vi "RS_RTO1024.vi"(4 "error in":T12, 7 "Command":string) -> (0 "error out":T12, 3 "Response":T10)   [LabVIEW 2018]
uses:
  MOKO_LabViewLibrary/MokoLowLevel/MokoLowLovelControl/MLLC_Error.ctl
  MOKO_LabViewLibrary/MokoLowLevel/MokoLowLovelControl/MLLC_Mode.ctl
  MOKO_LabViewLibrary/MokoLowLevel/MokoLowLovelControl/MLLC_Response.ctl
  MOKO_LabViewLibrary/MokoLowLevel/MokoLowLovelControl/MLLC_ConnectCluster.ctl
  MOKO_LabViewLibrary/MokoLowLevel/MokoLowLovelControl/MLLC_InterfaceType.ctl
  MOKO_LabViewLibrary/MokoLowLevel/MokoLowLovelControl/MLLC_OpenedSession.ctl
  MOKO_LabViewLibrary/MokoLowLevel/MokoLowLovelControl/MLLC_InterfaceSettings.ctl
  MOKO_LabViewLibrary/MokoLowLevel/MokoLowLovelControl/MLLC_InterfaceKind.ctl
  MOKO_LabViewLibrary/MokoLowLevel/MokoLowLovelControl/MLLC_DriverName.ctl
  MOKO_LabViewLibrary/MokoLowLevel/MokoLowLovelControl/MLLC_ErrorCode.ctl
  MOKO_LabViewLibrary/MokoLowLevel/MokoLowLovelControl/MLLC_ResponseInit.ctl
  MOKO_LabViewLibrary/MokoLowLevel/MokoLowLovelControl/MLLC_Request.ctl
  MOKO_LabViewLibrary/MokoLowLevel/MokoLowLovelControl/MLLC_Delay.ctl
panel:
  in  "Request":T1="*IDN?"
  in  "Response Init":T2="Rohde&Schwarz,FSW"
  in  "Error Code":T3=5450
  in  "Driver Name":T4="RS_RTO1024"
  in  "Settings":cluster{"Connect":T5}={"Connect"={"InterfaceType"=enum."VISA", "OpenedSession"="COM1", "InterfaceSettings"={"Interface"=enum."RS232", "EOS 4 read"=enum."LF (\\n)", "EOS 4 write"=enum."LF (\\n)", "TMO, ms"=10000, "Sett"=variant(cluster{"Baud Rate":u32, "Data Bits":u16, "Parity":u16, "Stop Bits":u16, "Flow Control":u16, "Eho":bool} {"Baud Rate"=75, "Data Bits"=0, "Parity"=0, "Stop Bits"=0, "Flow Control"=0, "Eho"=FALSE})}}}
  in  "Mode":T11=enum."Check"
  # "RS_RTO1024"
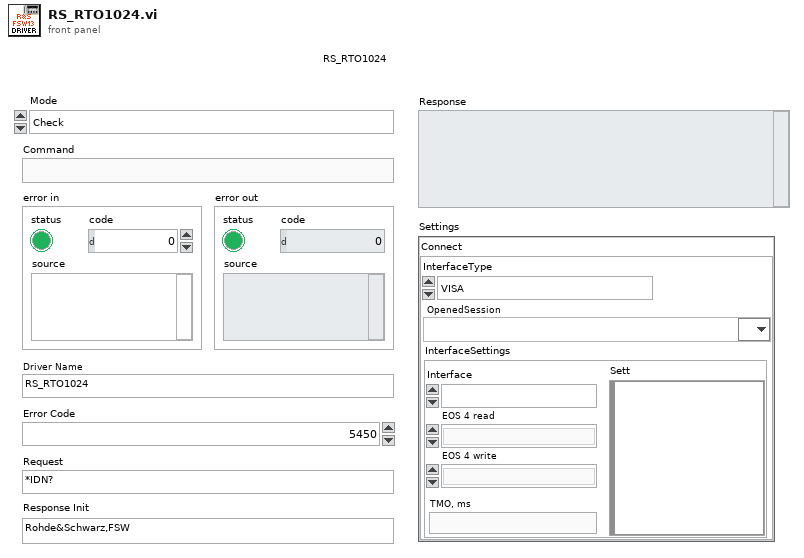
[diagram p1: front panel]
types:
  T1 = typedef "MLLC_Request.ctl" = string
  T2 = typedef "MLLC_ResponseInit.ctl" = string
  T3 = typedef "MLLC_ErrorCode.ctl" = u32
  T4 = typedef "MLLC_DriverName.ctl" = string
  T5 = typedef "MLLC_ConnectCluster.ctl" = cluster{"InterfaceType":T6, "OpenedSession":T7, "InterfaceSettings":T8}
  T6 = typedef "MLLC_InterfaceType.ctl" = enum16{"VISA", "Prologix USB-GPIB"}
  T7 = typedef "MLLC_OpenedSession.ctl" = refnum<visa-resource-name>
  T8 = typedef "MLLC_InterfaceSettings.ctl" = cluster{"Interface":T9, "EOS 4 read":enum16{"Default (=EOS 4 write)", "CR (\\r)", "LF (\\n)", "None"}, "EOS 4 write":enum16{"CR+LF (\\r\\n)", "CR (\\r)", "LF (\\n)", "None"}, "TMO, ms":i32, "Sett":variant}
  T9 = typedef "MLLC_InterfaceKind.ctl" = enum16{"RS232", "GPIB", "USB", "Ethernet", "another"}
  T10 = typedef "MLLC_Response.ctl" = string
  T11 = typedef "MLLC_Mode.ctl" = enum16{"get", "set", "close", "Init", "Check"}
  T12 = typedef "MLLC_Error.ctl" = errorcluster
  T13 = typedef "MLLC_Delay.ctl" = dbl
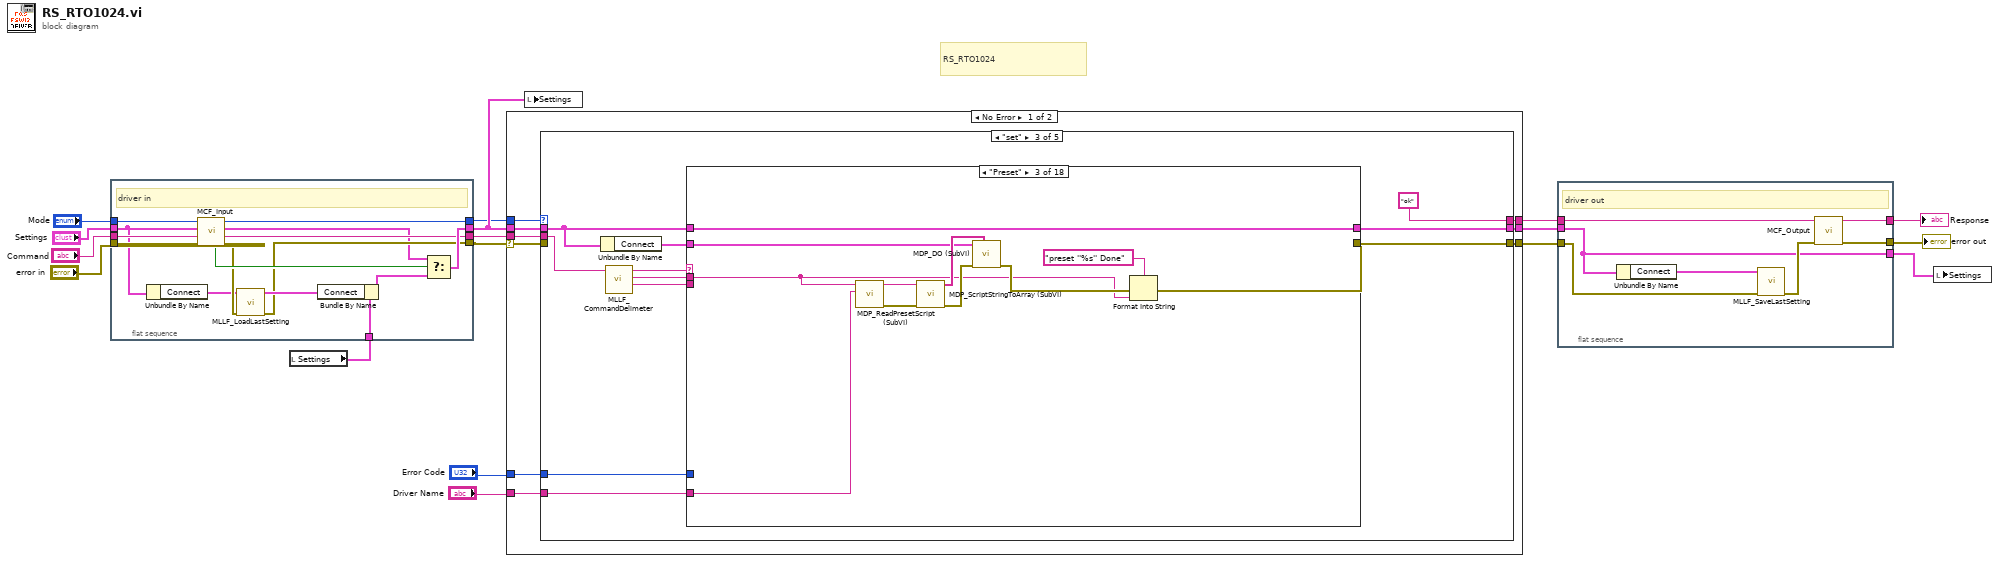
[diagram p0: block diagram]
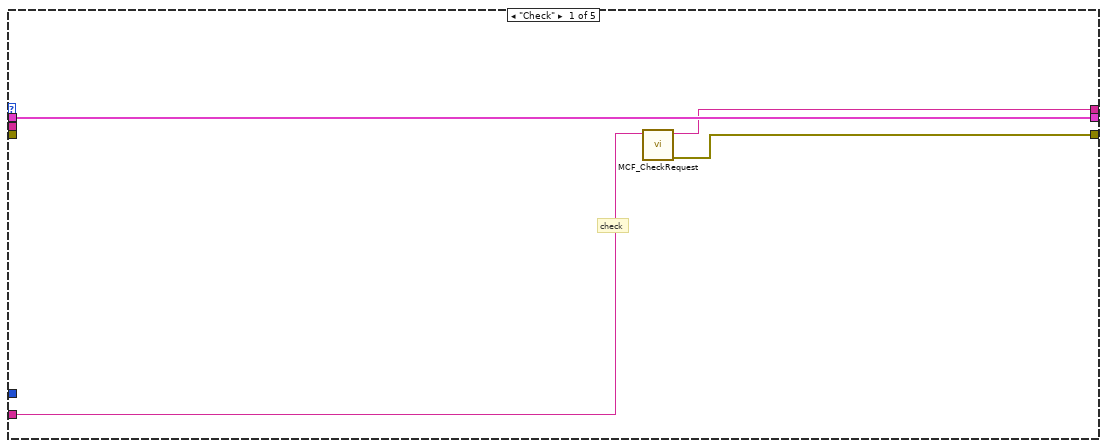
[diagram p2: hidden frame]
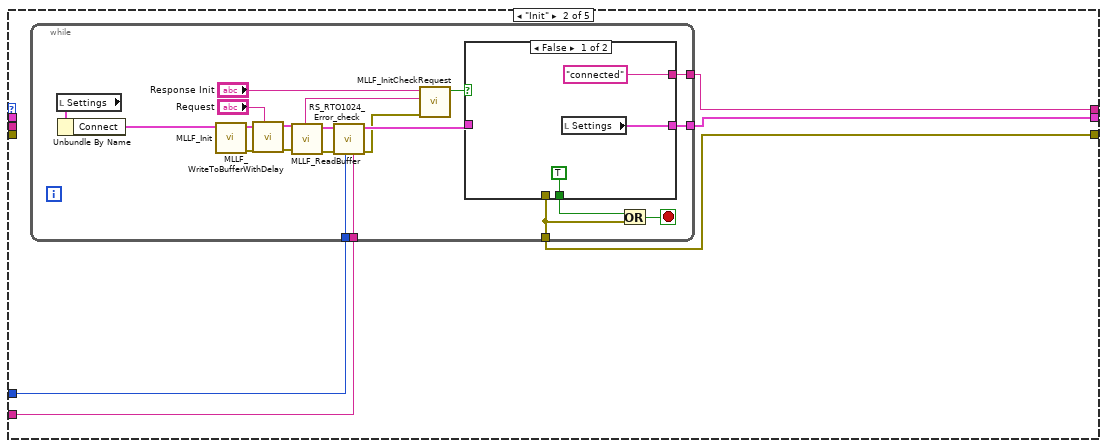
[diagram p3: hidden frame]
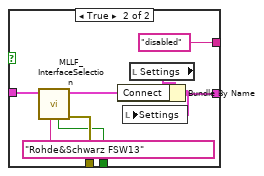
[diagram p4: hidden frame]
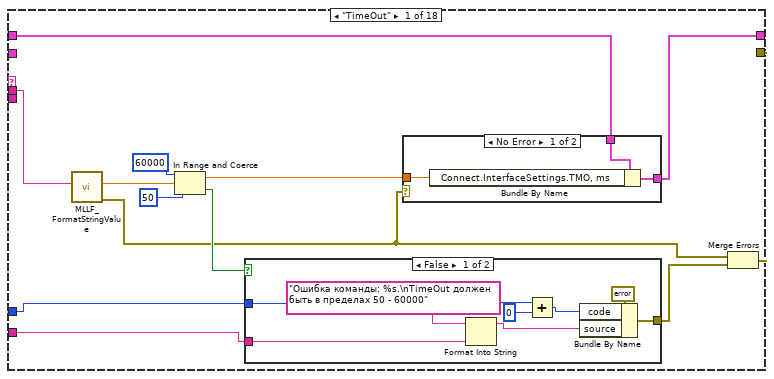
[diagram p5: hidden frame]
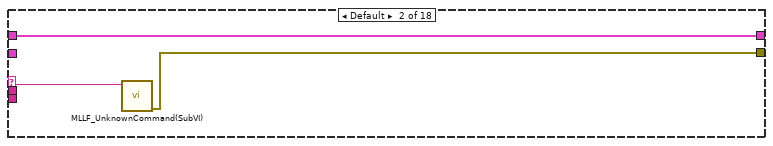
[diagram p8: hidden frame]
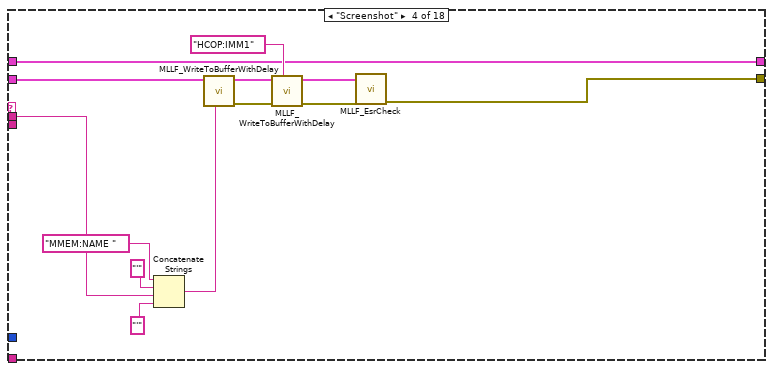
[diagram p9: hidden frame]
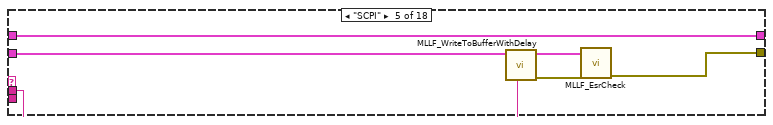
[diagram p10: hidden frame]
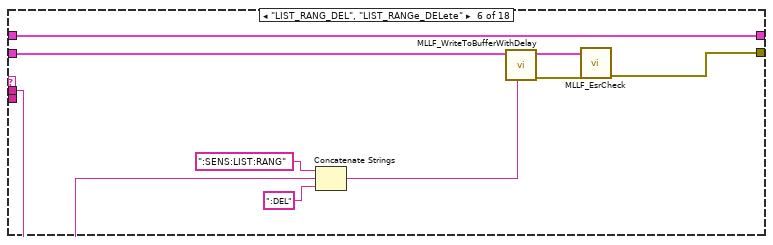
[diagram p11: hidden frame]
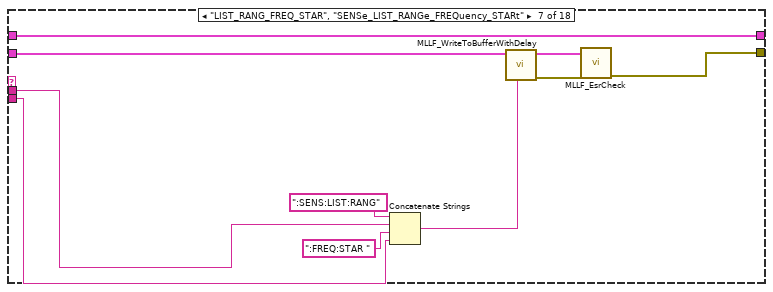
[diagram p12: hidden frame]
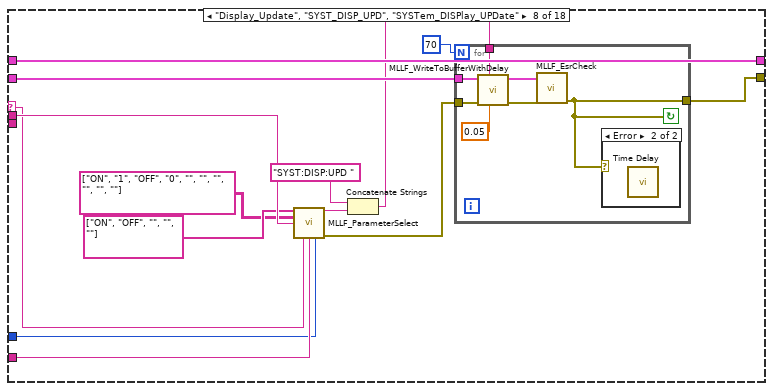
[diagram p13: hidden frame]
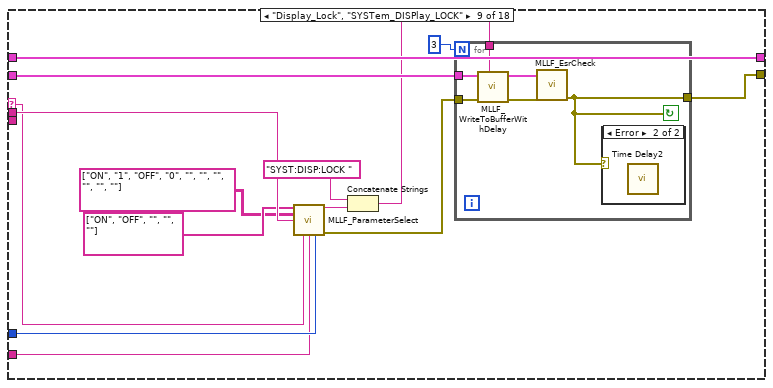
[diagram p15: hidden frame]
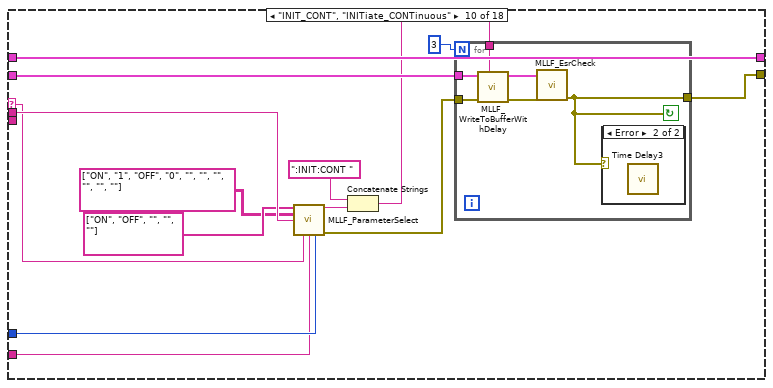
[diagram p17: hidden frame]
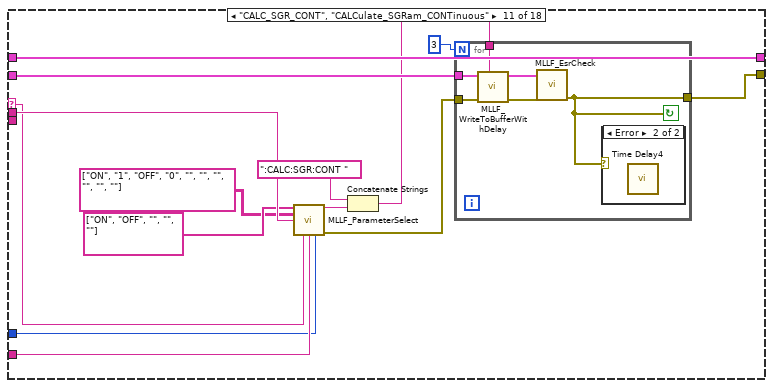
[diagram p19: hidden frame]
diagram:
  # "RS_RTO1024"
  n1 = flat-sequence {
    tunnel: [w22] -> w7
    tunnel: [w24] -> w8
    tunnel: "Command" -> [w25]
    tunnel: "Mode" -> [w27]
    tunnel: "Settings" -> [w19]
    tunnel: [w29] -> w10
    tunnel: w11 -> [w28]
    tunnel: "error in" -> [w21]
    tunnel: [w20] -> w9
    frame #0 {
      # "driver in"
      n2 = Unbundle By Name(w19) -> ("Connect"=w18:T5)
      n3 = call "MCF_Input.vi"("Error In"=w21, "Command in"=w25, "Mode in"=w27) -> ("Error Out"=w23:errorcluster, "Command out"=w24:string, "Mode out"=w20:T11, "Boolean"=w26:bool)  [unwired: 5 in]
      n4 = call "MLLF_LoadLastSetting.vi"("Error In"=w23, "DriverConnectCluster in"=w18) -> ("Error Out"=w22:errorcluster, "DriverConnectCluster out"=w30:T5)  [unwired: 8 in]
      n5 = Bundle By Name(cluster=w28, "Connect"=w30) -> (w31:cluster{"Connect":T5})
      n6 = Select(t=w19, s=w26, f=w31) -> (s? t:f=w29:cluster{"Connect":T5})
    }
  }
  n7 = local read "Settings"() -> (w11:cluster{"Connect":T5})
  n8 = case shown="No Error" w7 {
    selector: w7 -> [w36 w402]
    tunnel: [w38 w402] -> w1
    tunnel: w9 -> [w40 _]
    tunnel: [w39 "error" ("Output String")] -> w6
    tunnel: w8 -> [w37 _]
    tunnel: w10 -> [w33 w401]
    tunnel: "Error Code" -> [w35 _]
    tunnel: "Driver Name" -> [w34 _]
    tunnel: [w32 w401] -> w2
    frame No Error {
      n9 = case shown="\"set\"" w40 {
        tunnel: [w42 w47 "ok" ("Output String") w322 "close" ("Output String")] -> w39
        tunnel: [w41 w46 w85 w325 w398] -> w38
        tunnel: w37 -> [_ _ w92 w331 _]
        tunnel: w36 -> [_ _ _ _ _]
        tunnel: w35 -> [_ w49 w91 w328 _]
        tunnel: w34 -> [w43 w48 w88 w327 _]
        tunnel: w33 -> [w44 _ w90 w330 w397]
        tunnel: [w44 w45 w89 w329 w397] -> w32
        frame "Check" {
          # "check"
          # "Проверка подленности пользователя в соответствии с протоколом MD5."
          n10 = call "MCF_CheckRequest.vi"("Driver Name"=w43) -> ("Error Out"=w41:errorcluster, "Output String"=w42:string)  [unwired: 9 in]
        }
        frame "Init" {
          # "Тут проходит инициализация оборудования"
          n11 = while {
            tunnel: [w63] -> w46
            tunnel: w49 -> [w60]
            tunnel: w48 -> [w59]
            tunnel: [w55] -> w47
            tunnel: [w56] -> w45
            stop <- w62 stop-if-true
            n12 = local read "Settings"() -> (w66:cluster{"Connect":T5})
            n13 = Unbundle By Name(w66) -> ("Connect"=w52:T5)
            n14 = call "MLLF_Init.vi"("DriverConnect in"=w52) -> ("Error Out"=w68:errorcluster, "DriverConnect out"=w67:T5)  [unwired: 7 in]
            n15 = call "MLLF_WriteToBufferWithDelay.vi"("Command"="Request", "Error In"=w68, "DriverConnect in"=w67) -> ("Error Out"=w70:errorcluster, "DriverConnect out"=w69:T5)  [unwired: 7 in]
            n16 = call "MLLF_ReadBuffer.vi"("Error In"=w70, "DriverConnect in"=w69) -> ("Error Out"=w57:errorcluster, "DriverConnect out"=w58:T5, "String"=w54:string)  [unwired: 6 in]
            n17 = call "RS_RTO1024_Error_check.vi"("Driver Name"=w59, "Error Code"=w60, "error in"=w57, "DriverConnect in"=w58) -> ("error out"=w51:T12, "DriverConnect out"=w61:T5)  [unwired: 6 in]
            n18 = call "MLLF_InitCheckRequest.vi"("error in (no error)"=w51, "Answer"=w54, "Response Init"="Response Init") -> ("Design"=w50:bool)  [unwired: 5 in, 3 out]
            n19 = case shown="False" w50 {
              tunnel: w61 -> [_ w80]
              tunnel: [TRUE w74] -> w64
              tunnel: [_ w81] -> w63
              tunnel: [w72 w76] -> w56
              tunnel: ["connected" "disabled"] -> w55
              frame False {
                n20 = local read "Settings"() -> (w72:cluster{"Connect":T5})
              }
              frame True {
                n21 = call "MLLF_InterfaceSelection.vi"("Driver Name"="Rohde&Schwarz FSW13" ("String"), "DriverConnect in"=w80) -> ("error out"=w81:T12, "DriverConnect out"=w78:T5, "stop init?"=w74:bool)  [unwired: 5 in, 2 out]
                n22 = local read "Settings"() -> (w77:cluster{"Connect":T5})
                n23 = Bundle By Name(cluster=w77, "Connect"=w78) -> (w76:cluster{"Connect":T5})
                n24 = local write "Settings"(w76) -> ()
              }
            }
            n25 = Or(x=w64, y=w63) -> (x .or. y?=w62:bool)
          }
        }
        frame "set" {
          # "Тут реализованы функции DriverSet"
          n26 = Unbundle By Name(w90) -> ("Connect"=w86:T5)
          n27 = call "MLLF_CommandDelimeter.vi"("command with param"=w92) -> ("param 2"=w82:string, "param 1"=w83:string, "command"=w84:string)  [unwired: 6 in, 2 out]
          n28 = case shown="\"Preset\"" w84 {
            selector: w84 -> [_ w119 _ _ _ _ _ w170 w191 w211 w231 w251 _ _ _ _ _ _]
            tunnel: w90 -> [w95 w120 w121 w136 w149 w158 w168 w183 w204 w224 w244 w264 w275 w285 w299 w308 w314 w321]
            tunnel: [w94 w120 w121 w136 w149 w158 w168 w183 w204 w224 w244 w264 w275 w285 w299 w308 w314 w321] -> w89
            tunnel: w83 -> [w93 _ w124 w135 w147 w152 w161 w180 w201 w221 w241 w261 _ _ w292 _ _ _]
            tunnel: w91 -> [w97 _ _ _ _ _ _ w171 w193 w213 w232 w253 _ _ _ _ _ _]
            tunnel: w88 -> [w98 _ w123 _ _ _ _ w172 w192 w212 w233 w252 _ _ _ _ _ _]
            tunnel: [w96 w118 w122 w132 w148 w157 w167 w182 w203 w223 w243 w263 w274 w284 w298 w307 w313 w320] -> w85
            tunnel: w86 -> [_ _ w125 w144 w150 w159 w169 w181 w202 w222 w242 w262 w273 w283 w297 w306 w312 w319]
            tunnel: w82 -> [_ _ _ _ _ _ w160 _ _ _ _ _ _ _ w291 _ _ _]
            frame "TimeOut" {
              n29 = call "MLLF_FormatStringValue.vi"("String Value"=w93) -> ("error out"=w100:T12, "number"=w99:dbl)  [unwired: 8 in, 1 out]
              n30 = In Range and Coerce(upper limit=60000, x=w99, lower limit=50) -> (coerced(x)=w103:dbl, In Range?=w101:bool)
              n31 = case shown="False" w101 {
                tunnel: [w112 _] -> w102
                tunnel: w97 -> [w111 _]
                tunnel: w98 -> [w110 _]
                frame False {
                  n32 = Format Into String(format string="Ошибка команды: %s.\nTimeOut должен быть в пределах 50 - 60000", w110) -> (resulting string=w114:string)  [unwired: 2 in, 1 out]
                  n33 = Add(x=w111, y=0) -> (x+y=w115:T3)
                  n34 = Bundle By Name(cluster=errorcluster {"status"=TRUE, "code"=0, "source"=""} ("error out"), "code"=w115, "source"=w114) -> (w112:errorcluster)
                }
                frame True {
                }
              }
              n35 = case shown="No Error" w100 {
                tunnel: [w108 w109] -> w94
                tunnel: w95 -> [w107 w109]
                tunnel: w103 -> [w106 _]
                frame No Error {
                  n36 = Bundle By Name(cluster=w107, "Connect.InterfaceSettings.TMO, ms"=w106) -> (w108:cluster{"Connect":T5})
                }
                frame Error {
                }
              }
              n37 = Merge Errors(w100, w102) -> (w96:errorcluster)
            }
            frame Default {
              n38 = call "MLLF_UnknownCommand(SubVI).vi"("Unknown command"=w119) -> ("error out"=w118:errorcluster)  [unwired: 10 in]
            }
            frame "Preset" {
              n39 = call "MDP_ReadPresetScript (SubVI).vi"("Driver Name"=w123, "String in"=w124) -> ("Error Out"=w129:errorcluster, "String out"=w130:string)  [unwired: 8 in]
              n40 = call "MDP_ScriptStringToArray (SubVI).vi"("Error In"=w129, "String script"=w130) -> ("Error Out"=w131:errorcluster, "Array script"=w126:string[])  [unwired: 8 in]
              n41 = call "MDP_DO (SubVI).vi"("Array script"=w126, "Error in (no error)"=w131, "DriverConnect in"=w125) -> ("Error Out"=w127:errorcluster)  [unwired: 7 in, 1 out]
              n42 = Format Into String(format string="preset ''%s'' Done" ("Befor substring"), error in=w127, w124) -> (error out=w122:errorcluster)  [unwired: 1 in, 1 out]
            }
            frame "Screenshot" {
              n43 = Concatenate Strings("MMEM:NAME " ("String"), "'" ("string"), w135, "'" ("string")) -> (w139:string)
              n44 = call "MLLF_WriteToBufferWithDelay.vi"("Command"=w139, "DriverConnect in"=w144) -> ("Error Out"=w138:errorcluster, "DriverConnect out"=w143:T5)  [unwired: 8 in]
              n45 = call "MLLF_WriteToBufferWithDelay.vi"("Command"="HCOP:IMM1" ("String"), "Error In"=w138, "DriverConnect in"=w143) -> ("Error Out"=w134:errorcluster, "DriverConnect out"=w133:T5)  [unwired: 7 in]
              n46 = call "MLLF_EsrCheck.vi"("error in"=w134, "DriverConnect in"=w133) -> ("error out"=w132:T12)  [unwired: 8 in, 1 out]
            }
            frame "SCPI" {
              n47 = call "MLLF_WriteToBufferWithDelay.vi"("Command"=w147, "DriverConnect in"=w150) -> ("Error Out"=w145:errorcluster, "DriverConnect out"=w146:T5)  [unwired: 8 in]
              n48 = call "MLLF_EsrCheck.vi"("error in"=w145, "DriverConnect in"=w146) -> ("error out"=w148:T12)  [unwired: 8 in, 1 out]
            }
            frame "LIST_RANG_DEL", "LIST_RANGe_DELete" {
              n49 = Concatenate Strings(":SENS:LIST:RANG" ("String"), w152, ":DEL" ("string")) -> (w151:string)
              n50 = call "MLLF_WriteToBufferWithDelay.vi"("Command"=w151, "DriverConnect in"=w159) -> ("Error Out"=w155:errorcluster, "DriverConnect out"=w156:T5)  [unwired: 8 in]
              n51 = call "MLLF_EsrCheck.vi"("error in"=w155, "DriverConnect in"=w156) -> ("error out"=w157:T12)  [unwired: 8 in, 1 out]
            }
            frame "LIST_RANG_FREQ_STAR", "SENSe_LIST_RANGe_FREQuency_STARt" {
              n52 = Concatenate Strings(":SENS:LIST:RANG" ("String"), w161, ":FREQ:STAR " ("string"), w160) -> (w162:string)
              n53 = call "MLLF_WriteToBufferWithDelay.vi"("Command"=w162, "DriverConnect in"=w169) -> ("Error Out"=w165:errorcluster, "DriverConnect out"=w166:T5)  [unwired: 8 in]
              n54 = call "MLLF_EsrCheck.vi"("error in"=w165, "DriverConnect in"=w166) -> ("error out"=w167:T12)  [unwired: 8 in, 1 out]
            }
            frame "Display_Update", "SYST_DISP_UPD", "SYSTem_DISPlay_UPDate" {
              n55 = call "MLLF_ParameterSelect.vi"("Command to equipment"=string[] ["ON", "OFF", "", "", ""], "Names"=string[][] [["ON", "1"], ["OFF", "0"], ["", ""], ["", ""], ["", ""]], "Input"=w180, "Command"=w170, "Driver Name"=w172, "Error Code"=w171) -> ("Choice"=w176:string, "Error Out"=w173:errorcluster)  [unwired: 8 in]
              n56 = Concatenate Strings("SYST:DISP:UPD " ("string"), w176) -> (w175:string)
              n57 = for {
                N: 70 -> [_]
                tunnel: [w185] -> w182
                tunnel: w181 -> [w188]
                tunnel: w175 -> [w187]
                tunnel: w173 -> [w186]
                stop <- w185 continue-if-true
                n58 = call "MLLF_WriteToBufferWithDelay.vi"("Delay Time ( 0,05 s)"=T13 0.05, "Command"=w187, "Error In"=w186, "DriverConnect in"=w188) -> ("Error Out"=w190:errorcluster, "DriverConnect out"=w189:T5)  [unwired: 6 in]
                n59 = call "MLLF_EsrCheck.vi"("error in"=w190, "DriverConnect in"=w189) -> ("error out"=w185:T12)  [unwired: 8 in, 1 out]
                n60 = case shown="Error" w185 {
                  frame No Error {
                  }
                  frame Error {
                    n61 = call "Time Delay"() -> ()  [unwired: 11 in, 1 out]
                  }
                }
              }
            }
            frame "Display_Lock", "SYSTem_DISPlay_LOCK" {
              n62 = call "MLLF_ParameterSelect.vi"("Command to equipment"=string[] ["ON", "OFF", "", "", ""], "Names"=string[][] [["ON", "1"], ["OFF", "0"], ["", ""], ["", ""], ["", ""]], "Input"=w201, "Command"=w191, "Driver Name"=w192, "Error Code"=w193) -> ("Choice"=w197:string, "Error Out"=w194:errorcluster)  [unwired: 8 in]
              n63 = Concatenate Strings("SYST:DISP:LOCK " ("string"), w197) -> (w196:string)
              n64 = for {
                N: 3 -> [_]
                tunnel: [w205] -> w203
                tunnel: w202 -> [w208]
                tunnel: w196 -> [w207]
                tunnel: w194 -> [w206]
                stop <- w205 continue-if-true
                n65 = call "MLLF_WriteToBufferWithDelay.vi"("Command"=w207, "Error In"=w206, "DriverConnect in"=w208) -> ("Error Out"=w210:errorcluster, "DriverConnect out"=w209:T5)  [unwired: 7 in]
                n66 = call "MLLF_EsrCheck.vi"("error in"=w210, "DriverConnect in"=w209) -> ("error out"=w205:T12)  [unwired: 8 in, 1 out]
                n67 = case shown="Error" w205 {
                  frame No Error {
                  }
                  frame Error {
                    n68 = call "Time Delay2"() -> ()  [unwired: 11 in, 1 out]
                  }
                }
              }
            }
            frame "INIT_CONT", "INITiate_CONTinuous" {
              n69 = call "MLLF_ParameterSelect.vi"("Command to equipment"=string[] ["ON", "OFF", "", "", ""], "Names"=string[][] [["ON", "1"], ["OFF", "0"], ["", ""], ["", ""], ["", ""]], "Input"=w221, "Command"=w211, "Driver Name"=w212, "Error Code"=w213) -> ("Choice"=w217:string, "Error Out"=w214:errorcluster)  [unwired: 8 in]
              n70 = Concatenate Strings(":INIT:CONT " ("string"), w217) -> (w216:string)
              n71 = for {
                N: 3 -> [_]
                tunnel: [w225] -> w223
                tunnel: w222 -> [w228]
                tunnel: w216 -> [w227]
                tunnel: w214 -> [w226]
                stop <- w225 continue-if-true
                n72 = call "MLLF_WriteToBufferWithDelay.vi"("Command"=w227, "Error In"=w226, "DriverConnect in"=w228) -> ("Error Out"=w230:errorcluster, "DriverConnect out"=w229:T5)  [unwired: 7 in]
                n73 = call "MLLF_EsrCheck.vi"("error in"=w230, "DriverConnect in"=w229) -> ("error out"=w225:T12)  [unwired: 8 in, 1 out]
                n74 = case shown="Error" w225 {
                  frame No Error {
                  }
                  frame Error {
                    n75 = call "Time Delay3"() -> ()  [unwired: 11 in, 1 out]
                  }
                }
              }
            }
            frame "CALC_SGR_CONT", "CALCulate_SGRam_CONTinuous" {
              n76 = call "MLLF_ParameterSelect.vi"("Command to equipment"=string[] ["ON", "OFF", "", "", ""], "Names"=string[][] [["ON", "1"], ["OFF", "0"], ["", ""], ["", ""], ["", ""]], "Input"=w241, "Command"=w231, "Driver Name"=w233, "Error Code"=w232) -> ("Choice"=w237:string, "Error Out"=w234:errorcluster)  [unwired: 8 in]
              n77 = Concatenate Strings(":CALC:SGR:CONT " ("string"), w237) -> (w236:string)
              n78 = for {
                N: 3 -> [_]
                tunnel: [w245] -> w243
                tunnel: w242 -> [w248]
                tunnel: w236 -> [w247]
                tunnel: w234 -> [w246]
                stop <- w245 continue-if-true
                n79 = call "MLLF_WriteToBufferWithDelay.vi"("Command"=w247, "Error In"=w246, "DriverConnect in"=w248) -> ("Error Out"=w250:errorcluster, "DriverConnect out"=w249:T5)  [unwired: 7 in]
                n80 = call "MLLF_EsrCheck.vi"("error in"=w250, "DriverConnect in"=w249) -> ("error out"=w245:T12)  [unwired: 8 in, 1 out]
                n81 = case shown="Error" w245 {
                  frame No Error {
                  }
                  frame Error {
                    n82 = call "Time Delay4"() -> ()  [unwired: 11 in, 1 out]
                  }
                }
              }
            }
            frame "CALC_SPEC_CONT", "CALCulate_SPECtrogram_CONTinuous" {
              n83 = call "MLLF_ParameterSelect.vi"("Command to equipment"=string[] ["ON", "OFF", "", "", ""], "Names"=string[][] [["ON", "1"], ["OFF", "0"], ["", ""], ["", ""], ["", ""]], "Input"=w261, "Command"=w251, "Driver Name"=w252, "Error Code"=w253) -> ("Choice"=w257:string, "Error Out"=w254:errorcluster)  [unwired: 8 in]
              n84 = Concatenate Strings(":CALC:SPEC:CONT " ("string"), w257) -> (w256:string)
              n85 = for {
                N: 3 -> [_]
                tunnel: [w265] -> w263
                tunnel: w262 -> [w268]
                tunnel: w256 -> [w267]
                tunnel: w254 -> [w266]
                stop <- w265 continue-if-true
                n86 = call "MLLF_WriteToBufferWithDelay.vi"("Command"=w267, "Error In"=w266, "DriverConnect in"=w268) -> ("Error Out"=w270:errorcluster, "DriverConnect out"=w269:T5)  [unwired: 7 in]
                n87 = call "MLLF_EsrCheck.vi"("error in"=w270, "DriverConnect in"=w269) -> ("error out"=w265:T12)  [unwired: 8 in, 1 out]
                n88 = case shown="Error" w265 {
                  frame No Error {
                  }
                  frame Error {
                    n89 = call "Time Delay6"() -> ()  [unwired: 11 in, 1 out]
                  }
                }
              }
            }
            frame "CALC_SGR_CLE", "CALCulate_SGRam_CLEar" {
              n90 = for {
                N: 3 -> [_]
                tunnel: [w276] -> w274
                tunnel: w273 -> [w278]
                tunnel: "CALC:SGR:CLE" ("string") -> [w277]
                stop <- w276 continue-if-true
                n91 = call "MLLF_WriteToBufferWithDelay.vi"("Command"=w277, "DriverConnect in"=w278) -> ("Error Out"=w280:errorcluster, "DriverConnect out"=w279:T5)  [unwired: 8 in]
                n92 = call "MLLF_EsrCheck.vi"("error in"=w280, "DriverConnect in"=w279) -> ("error out"=w276:T12)  [unwired: 8 in, 1 out]
                n93 = case shown="Error" w276 {
                  frame No Error {
                  }
                  frame Error {
                    n94 = call "Time Delay7"() -> ()  [unwired: 11 in, 1 out]
                  }
                }
              }
            }
            frame "CALC_SPEC_CLE", "CALCulate_SPECtrogram_CLEar" {
              n95 = for {
                N: 3 -> [_]
                tunnel: [w286] -> w284
                tunnel: w283 -> [w288]
                tunnel: "CALC:SPEC:CLE" ("string") -> [w287]
                stop <- w286 continue-if-true
                n96 = call "MLLF_WriteToBufferWithDelay.vi"("Command"=w287, "DriverConnect in"=w288) -> ("Error Out"=w290:errorcluster, "DriverConnect out"=w289:T5)  [unwired: 8 in]
                n97 = call "MLLF_EsrCheck.vi"("error in"=w290, "DriverConnect in"=w289) -> ("error out"=w286:T12)  [unwired: 8 in, 1 out]
                n98 = case shown="Error" w286 {
                  frame No Error {
                  }
                  frame Error {
                    n99 = call "Time Delay8"() -> ()  [unwired: 11 in, 1 out]
                  }
                }
              }
            }
            frame "INIT_OPC", "INITiate_OPC" {
              n100 = case shown="\"Timeout\", \"TMO\"" w292 {
                tunnel: w291 -> [_ w302]
                tunnel: [20.0 w301] -> w293
                frame "False", Default {
                }
                frame "Timeout", "TMO" {
                  n101 = Scan From String(input string=w302) -> (output 1=w301:dbl)  [unwired: 4 in, 3 out]
                }
              }
              n102 = call "MLLF_WriteToBufferWithDelay.vi"("Delay Time ( 0,05 s)"=w293, "Command"="INIT:SPUR" ("string"), "DriverConnect in"=w297) -> ("Error Out"=w295:errorcluster, "DriverConnect out"=w294:T5)  [unwired: 7 in]
              n103 = call "MLLF_EsrCheck.vi"("error in"=w295, "DriverConnect in"=w294) -> ("error out"=w298:T12)  [unwired: 8 in, 1 out]
            }
            frame "ListXAdj" {
              # ":SENS:LIST:XADJ;*WAI"
              n104 = call "MLLF_WriteToBufferWithDelay.vi"("Command"=":SENS:LIST:XADJ" ("string"), "DriverConnect in"=w306) -> ("Error Out"=w304:errorcluster, "DriverConnect out"=w303:T5)  [unwired: 8 in]
              n105 = call "MLLF_EsrCheck.vi"("error in"=w304, "DriverConnect in"=w303) -> ("error out"=w307:T12)  [unwired: 8 in, 1 out]
            }
            frame "SensAdjAll" {
              # ":SENS:ADJ:ALL;*WAI"
              n106 = call "MLLF_WriteToBufferWithDelay.vi"("Command"=":SENS:ADJ:ALL;*WAI" ("string"), "DriverConnect in"=w312) -> ("Error Out"=w310:errorcluster, "DriverConnect out"=w309:T5)  [unwired: 8 in]
              n107 = call "MLLF_EsrCheck.vi"("error in"=w310, "DriverConnect in"=w309) -> ("error out"=w313:T12)  [unwired: 8 in, 1 out]
            }
            frame "RESET", "RST" {
              n108 = call "MLLF_WriteToBufferWithDelay.vi"("Delay Time ( 0,05 s)"=20.0, "Command"="*RST" ("string"), "DriverConnect in"=w319) -> ("Error Out"=w317:errorcluster, "DriverConnect out"=w316:T5)  [unwired: 7 in]
              n109 = call "MLLF_EsrCheck.vi"("error in"=w317, "DriverConnect in"=w316) -> ("error out"=w320:T12)  [unwired: 8 in, 1 out]
            }
          }
        }
        frame "get" {
          # "Тут реализованы функции DriverGet"
          n110 = call "MLLF_CommandDelimeter.vi"("command with param"=w331) -> ("param 1"=w323:string, "command"=w324:string)  [unwired: 6 in, 3 out]
          n111 = Unbundle By Name(w330) -> ("Connect"=w326:T5)
          n112 = case shown="\"------ID-------\"" w324 {
            selector: w324 -> [w333 _ _ _ _ _ _]
            tunnel: [w332 _ _ w351 w365 w374 w381] -> w325
            tunnel: w328 -> [_ _ _ _ _ _ _]
            tunnel: [w336 w339 w340 w350 w364 w378 w395] -> w329
            tunnel: w330 -> [w336 w339 w340 w350 w364 w378 w395]
            tunnel: [w334 w337 _ _ _ _ _] -> _
            tunnel: w326 -> [_ _ _ w352 w366 w379 w390]
            tunnel: w327 -> [_ _ _ _ _ _ w383]
            tunnel: [_ _ _ w343 w360 w373 "write to Data.txt" ("output")] -> w322
            tunnel: w323 -> [_ _ _ _ _ w377 _]
            frame "False", Default {
              # "DEFAULT"
              n113 = call "MLLF_UnknownCommand(SubVI).vi"("Unknown command"=w333) -> ("error out"=w332:errorcluster)  [unwired: 10 in]
              n114 = Build Array(0 ("TimeOut")) -> (w334:i32[])
            }
            frame "TIMEOUT" {
              # "Время ожидания ответа от прибора."
              n115 = Unbundle By Name(w339) -> ("Connect.InterfaceSettings.TMO, ms"=w338:i32)
              n116 = Build Array(w338) -> (w337:i32[])
            }
            frame "------ID-------" {
            }
            frame "model" {
              n117 = call "RS_RTO1024_FASTQUERY.vi"("input"="*IDN?", "DriverConnect in"=w352) -> ("error out"=w351:T12, "output"=w349:string)  [unwired: 7 in, 1 out]
              n118 = for {
                N: 4 -> [_]
                shift-right: [w354] -> _
                shift-left: w349 -> [w357]
                tunnel: [w356] -> w348 mode=indexing
                stop <- w355 stop-if-true
                n119 = Match Pattern(string=w357, regular expression=",") -> (before substring=w356:string, after substring=w354:string)  [unwired: 1 in, 2 out]
                n120 = Empty String/Path?(string/path=w354) -> (empty?=w355:bool)
              }
              n121 = Index Array(array=w348, index #1=0 ("index"), index #2=1 ("index")) -> (element #1=w346:string, element #2=w344:string)
              n122 = Concatenate Strings(w346, " " ("string"), w344) -> (w343:string)
            }
            frame "FW", "ver", "version" {
              n123 = call "RS_RTO1024_FASTQUERY.vi"("input"="*IDN?", "DriverConnect in"=w366) -> ("error out"=w365:T12, "output"=w361:string)  [unwired: 7 in, 1 out]
              n124 = for {
                N: 4 -> [_]
                shift-right: [w368] -> _
                shift-left: w361 -> [w371]
                tunnel: [w370] -> w363 mode=indexing
                stop <- w369 stop-if-true
                n125 = Match Pattern(string=w371, regular expression=",") -> (before substring=w370:string, after substring=w368:string)  [unwired: 1 in, 2 out]
                n126 = Empty String/Path?(string/path=w368) -> (empty?=w369:bool)
              }
              n127 = Index Array(array=w363, index=3) -> (element=w360:string)
            }
            frame "SCPI" {
              n128 = call "RS_RTO1024_FASTQUERY.vi"("input"=w377, "DriverConnect in"=w379) -> ("error out"=w375:T12, "DriverConnect out"=w376:T5, "output"=w373:string)  [unwired: 7 in]
              n129 = call "MLLF_EsrCheck.vi"("error in"=w375, "DriverConnect in"=w376) -> ("error out"=w374:T12)  [unwired: 8 in, 1 out]
            }
            frame "TraceDataSpur" {
              # "TRAC:DATA? SPUR"
              n130 = call "MLLF_WriteToBuffer.vi"("String"="TRAC:DATA? SPUR", "DriverConnect in"=w390) -> ("error out"=w391:T12, "DriverConnect out"=w392:T5)  [unwired: 6 in]
              n131 = call "MLLF_ReadBuffer.vi"("Error In"=w391, "DriverConnect in"=w392) -> ("Error Out"=w388:errorcluster, "DriverConnect out"=w389:T5, "String"=w393:string)  [unwired: 6 in]
              n132 = call <vilib>:"Trim Whitespace.vi"("string"=w393) -> ("trimmed string"=w387:string)  [unwired: 1 in]
              n133 = call "MLLF_EsrCheck.vi"("error in"=w388, "DriverConnect in"=w389) -> ("error out"=w382:T12)  [unwired: 8 in, 1 out]
              n134 = call "RS_RTO1024_ConvIntoFormatString.vi"("Mode"=enum16{"Value", "Status"}."Value", "Error In"=w382, "input string"=w387) -> ("Error Out"=w385:errorcluster, "output"=w384:string)  [unwired: 7 in]
              n135 = call "RS_RTO1024_SAve to datafile (SubVI).vi"("Error In"=w385, "Driver Name"=w383, "output"=w384) -> ("error out"=w381:errorcluster)  [unwired: 8 in]
            }
          }
        }
        frame "close" {
          # "Завершение сессии"
          n136 = Unbundle By Name(w397) -> ("Connect.OpenedSession"=w399:T7)
          n137 = VISA Close(VISA resource name=w399) -> (error out=w398:errorcluster)  [unwired: 1 in]
        }
      }
    }
    frame Error {
    }
  }
  n138 = local write "Settings"(w10) -> ()
  n139 = flat-sequence {
    tunnel: [w409] -> w5
    tunnel: w6 -> [w408]
    tunnel: w1 -> [w403]
    tunnel: w2 -> [w404]
    tunnel: [w404] -> w3
    tunnel: [w405] -> w4
    frame #0 {
      # "driver out"
      n140 = Unbundle By Name(w404) -> ("Connect"=w407:T5)
      n141 = call "MLLF_SaveLastSetting.vi"("error in"=w403, "DriverConnectCluster in"=w407) -> ("error out"=w406:T12)  [unwired: 8 in, 1 out]
      n142 = call "MCF_Output.vi"("Error In"=w406, "Input"=w408) -> ("Error Out"=w405:errorcluster, "Output"=w409:string)  [unwired: 8 in]
    }
  }
  n143 = local write "Settings"(w3) -> ()
  "error out" <- w4
  "Response" <- w5
